vi "knownhosts.vi"() -> ()   [LabVIEW 2013]
doc: "Illustrates how to read a collection of host keys from file."
uses:
  libssh2/libssh2_knownhost.ctl
  libssh2/Host Key Refnum.ctl
  libssh2/libssh2_init_default.vi
  libssh2/libssh2.lvlib
panel:
  out "error out":errorcluster
  out "hosts added":i32
  out "known hosts":T1[](array[typedef])
  in  "filename":path
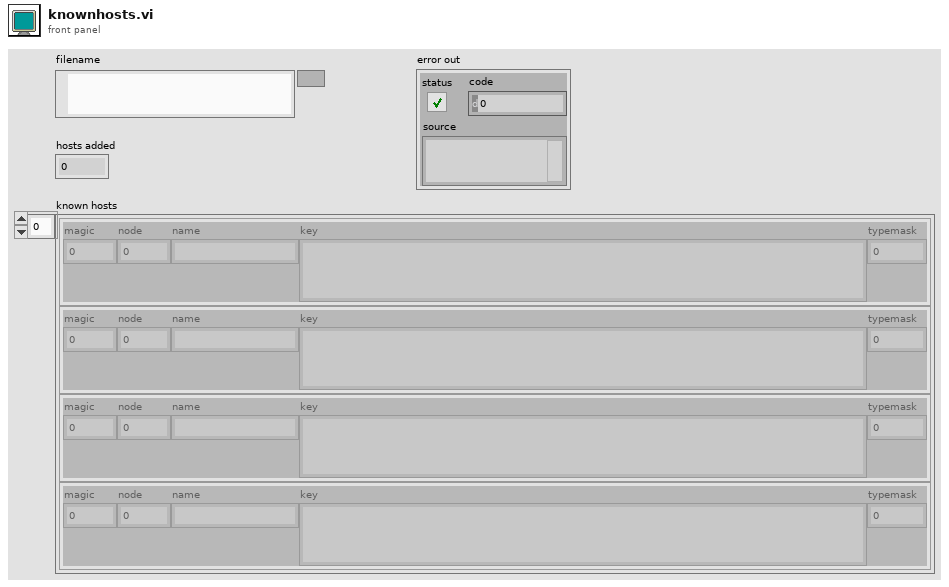
[diagram p1: front panel]
types:
  T1 = typedef "libssh2.lvlib/libssh2_knownhost.ctl" = cluster{"magic":u32, "node":u64, "name":string, "key":string, "typemask":i32}
  T2 = typedef "libssh2.lvlib/Host Key Refnum.ctl" = refnum<k1>
  T3 = typedef "libssh2.lvlib/Session Refnum.ctl" = refnum<k1>
  T4 = typedef "libssh2.lvlib/Host Key Database Refnum.ctl" = refnum<k1>
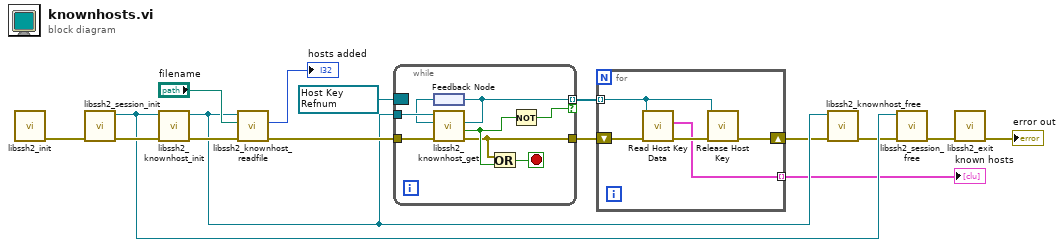
[diagram p0: block diagram]
diagram:
  w5 = T2 refnum items=["host key"] ("next")
  n1 = call-poly "libssh2_init.vi"() -> ("error out"=w16:errorcluster)  [unwired: 11 in]
  n2 = call "libssh2_session_init.vi"("error in (no error)"=w16) -> ("error out"=w15:errorcluster, "session"=w14:T3)  [unwired: 9 in]
  n3 = call "libssh2_knownhost_init.vi"("error in (no error)"=w15, "session"=w14) -> ("error out"=w11:errorcluster, "host key database"=w8:T4)  [unwired: 8 in]
  n4 = call "libssh2_knownhost_readfile.vi"("error in (no error)"=w11, "filename"="filename", "host key database"=w8) -> ("error out"=w10:errorcluster, "hosts added"=→"hosts added":i32)  [unwired: 7 in]
  n5 = while {
    tunnel: w10 -> [w24]
    tunnel: [w18] -> w7
    tunnel: w8 -> [w23]
    border: w5 -> [_]
    tunnel: [w20] -> w4 mode=indexing if=w17
    stop <- w22 stop-if-true
    n6 = feedback #1() -> (w21:T2)
    n7 = call "libssh2_knownhost_get.vi"("error in (no error)"=w24, "previous host key"=w21, "host key database"=w23) -> ("error out"=w18:errorcluster, "end reached"=w19:bool, "host key"=w20:T2)  [unwired: 6 in]
    n8 = feedback-in #1(w20) -> ()
    n9 = Or(x=w18, y=w19) -> (x .or. y?=w22:bool)
    n10 = Not(x=w19) -> (.not. x?=w17:bool)
  }
  n11 = for {
    shift-right: [w29] -> w6
    shift-left: w7 -> [w28]
    tunnel: w4 -> [w26] mode=indexing
    tunnel: [w25] -> w2 mode=indexing
    n12 = call "Read Host Key Data.vi"("error in (no error)"=w28, "host key"=w26) -> ("error out"=w27:errorcluster, "host key data"=w25:T1)  [unwired: 8 in]
    n13 = call "Release Host Key.vi"("error in (no error)"=w27, "host key"=w26) -> ("error out"=w29:errorcluster)  [unwired: 9 in]
  }
  "known hosts" <- w2
  n14 = call "libssh2_knownhost_free.vi"("error in (no error)"=w6, "host key database"=w8) -> ("error out"=w13:errorcluster)  [unwired: 9 in]
  n15 = call "libssh2_session_free.vi"("error in (no error)"=w13, "session"=w14) -> ("error out"=w12:errorcluster)  [unwired: 9 in]
  n16 = call "libssh2_exit.vi"("error in (no error)"=w12) -> ("error out"=→"error out":errorcluster)  [unwired: 10 in]
